vi "Actor Core.vi"(8 "error in":errorcluster, 11 "GameLogic in":refnum<class "GameLogic.lvclass">) -> (0 "error out":errorcluster, 3 "Actor out":refnum<class "Actor.lvclass">)   [LabVIEW 2019, in "GameLogic.lvlib" / "GameLogic.lvclass"]
doc: "(<B>Filename</B>: Actor Framework.lvlib:Actor.lvclass:Actor Core.vi)\n\nReceives messages to the actor, reacts to them, and initiates any error handling that may shut the actor down.\n\nDescendant classes may override this VI to append parallel tasks for the actor to complete while it handles messages. Overrides use the Call Parent Method node."
uses:
  GameLogic.lvclass
  C:/Program Files (x86)/National Instruments/LabVIEW 2019/vi.lib/ActorFramework/Actor/Actor.lvclass
  <vilib>/ActorFramework/Actor/Actor.lvclass
  <vilib>/ActorFramework/Actor/Actor.lvclass/Actor.ctl
  <vilib>/ActorFramework/Message Enqueuer/Message Enqueuer.lvclass/Message Enqueuer.ctl
  GameLogic.lvclass/GameLogic.ctl
  <vilib>/ActorFramework/Message Enqueuer/Init from Existing Queue.vi
  <vilib>/ActorFramework/Message Enqueuer/Enqueue.vi
  GameLogic Messages/Select Color to Display Msg/Select Color to Display Msg.lvclass
  C:/Program Files (x86)/National Instruments/LabVIEW 2019/vi.lib/ActorFramework/Message/Message.lvclass
  <vilib>/ActorFramework/Stop Msg/Stop Msg.lvclass
  <vilib>/ActorFramework/Message Priority Queue/Priority Enqueue.vi
  <vilib>/ActorFramework/Message Enqueuer/Message Enqueuer.lvclass
panel:
  out "Green":bool
  out "Yellow":bool
  out "Red":bool
  out "Blue":bool
  in  "Start":bool
  in  "stop":bool
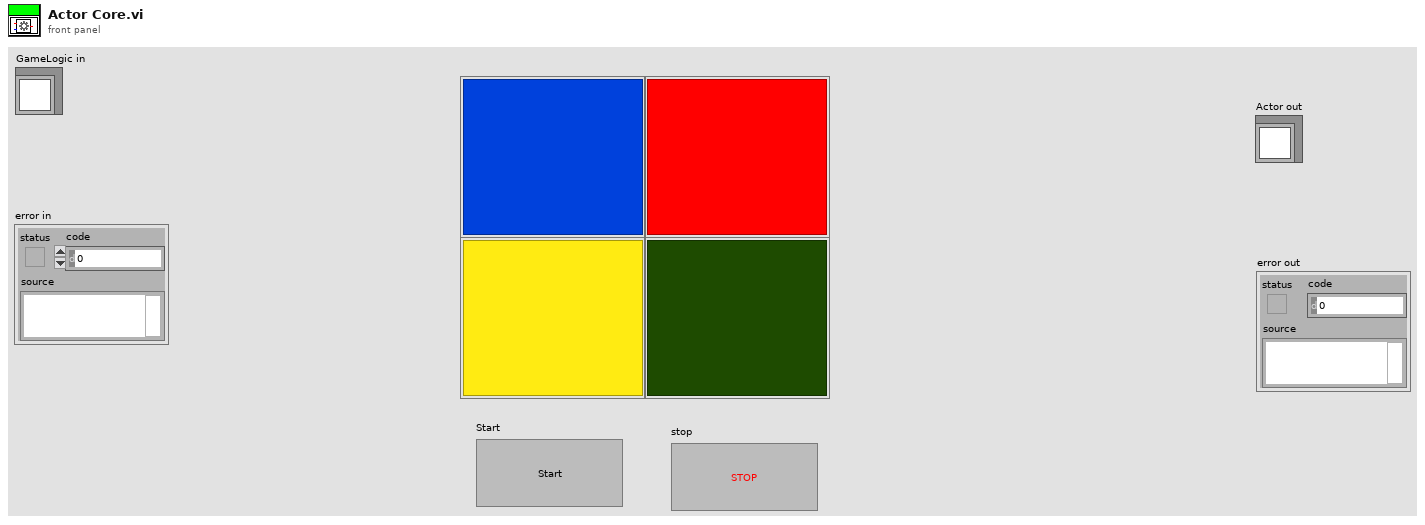
[diagram p1: front panel]
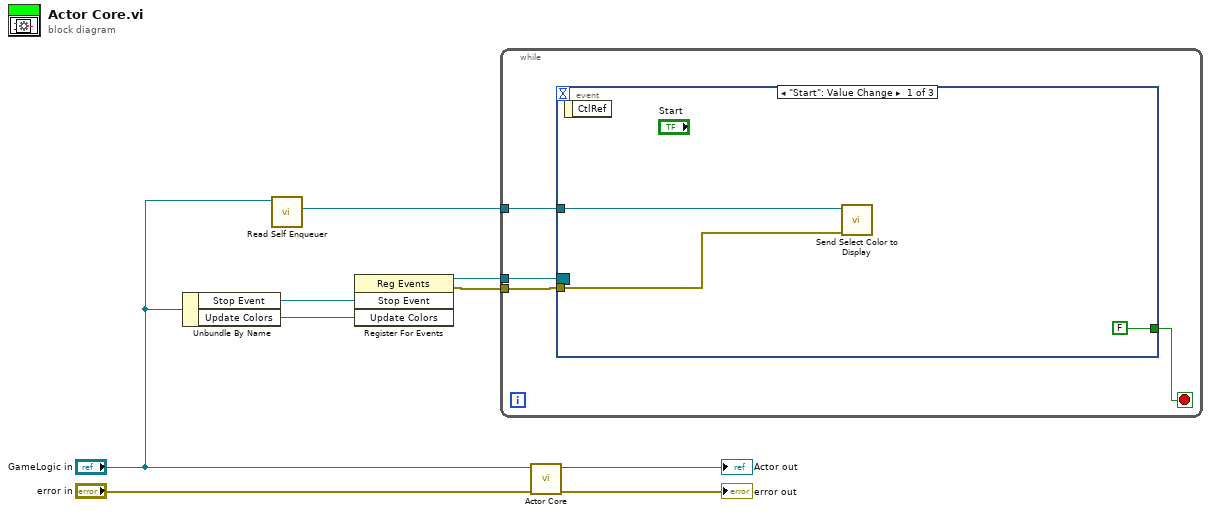
[diagram p0: block diagram]
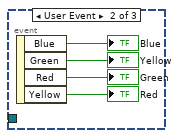
[diagram p2: hidden frame]
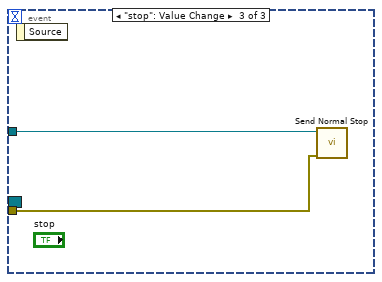
[diagram p3: hidden frame]
diagram:
  n1 = Unbundle By Name("GameLogic in") -> ("Stop Event"=w6:refnum<user-event>, "Update Colors"=w4:refnum<user-event>)
  n2 = call <vilib>:"Read Self Enqueuer.vi"("Actor"="GameLogic in") -> ("Self Enqueuer"=w2:refnum<class "Message Enqueuer.lvclass">)  [unwired: 10 in]
  n3 = register-events(w6, w4) -> (reference out=w3:refnum<event-registration>, error out=w1:errorcluster)  [unwired: 2 in]
  n4 = while {
    tunnel: w3 -> [w13]
    tunnel: w2 -> [w12]
    tunnel: w1 -> [w10]
    stop <- w11 stop-if-true
    n5 = event shown="[0] \"Start\": Value Change" {
      selector: w13 -> [_ _ _]
      dyn-events: _ -> [_ _ _]
      timeout: _ -> [_ _ _]
      tunnel: w12 -> [w15 _ w22]
      tunnel: [FALSE _ _] -> w11
      tunnel: w10 -> [w14 _ w21]
      event "Start": Value Change {
        n6 = event-data() -> ()  [unwired: 1 in, 1 out]
        n7 = call "Send Select Color to Display.vi"("error in (no error)"=w14, "Message Enqueuer"=w15) -> ()  [unwired: 8 in, 2 out]
      }
      event User Event {
        n8 = event-data() -> ("Blue"=→"Blue":bool, "Green"=→"Yellow":bool, "Red"=→"Green":bool, "Yellow"=→"Red":bool)  [unwired: 1 in]
      }
      event "stop": Value Change {
        n9 = event-data() -> ()  [unwired: 1 in, 1 out]
        n10 = call <vilib>:"Send Normal Stop.vi"("error in (no error)"=w21, "Message Enqueuer"=w22) -> ()  [unwired: 9 in, 1 out]
      }
    }
  }
  n11 = call-parent "Actor Core.vi"("error in"="error in", "Actor in"="GameLogic in") -> ("error out"=→"error out":errorcluster, "Actor out"=→"Actor out":refnum<class "Actor.lvclass">)  [unwired: 8 in]
